vi "Tektronix TTR500 Series Calibration.vi"(11 "VISA resource name":refnum<visa-resource-name>="TCPIP0::localhost::5026::SOCKET") -> (0 "error out":errorcluster, 3 "Trace":T1(graph))   [LabVIEW 2012]
uses:
  <instrlib>/Tektronix TTR500 Series/Tektronix TTR500 Series.lvlib
panel:
  in  "Measurement Parameters (S21)":u16(ring)=1 items=["S11", "S21", "S31", "S41", "S12", "S22", "S32", "S42", "S13", "S23", "S33", "S43", "S14", "S24", "S34", "S44", "A", "B", "C", "D", "R1", "R2", "R3", "R4", "AUX1", "AUX2", "TR", "T", "R"]
  in  "IF Bandwidth (10k [Hz])":dbl=10000.0 format="%#p"
  in  "Number of Measurement Points (201)":i32=201
  in  "Power Level (0)":dbl format="%#.3f"
  in  "Stop Frequency (4G [Hz])":dbl=4000000000.0 format="%#p"
  in  "Start Frequency (1G [Hz])":dbl=1000000000.0 format="%#p"
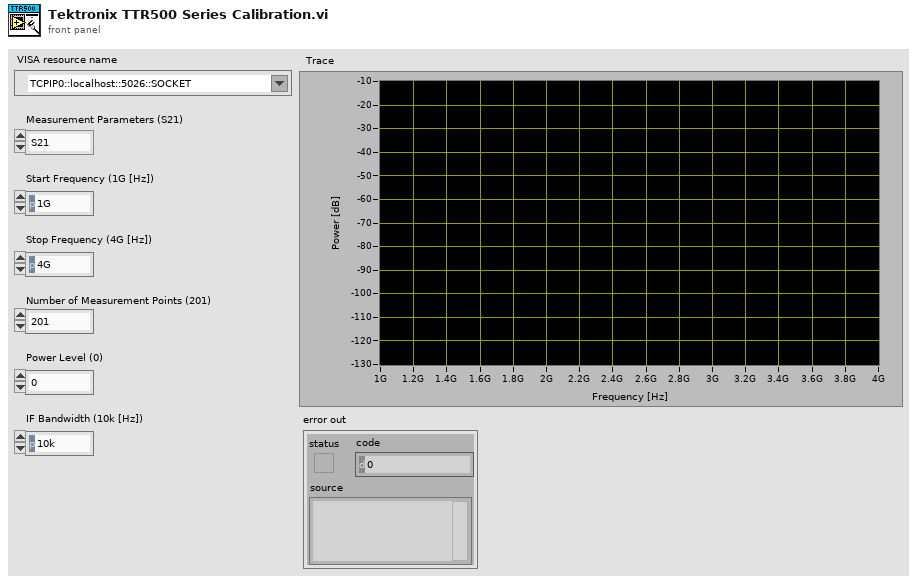
[diagram p1: front panel]
types:
  T1 = cluster{"Stimulus Data":dbl[], "Primary / Real":dbl[]}
  T2 = cluster{"Standard":u16, "Port 1 - response":i32, "Port 2 - stimulus":i32}[]
  T3 = enum16{"Open", "Short", "Load", "Through", "Isolation", "Gain Phase Open", "Gain Phase Short", "Gain Phase Load", "Gain Phase Through", "Gain Phase Isolation"}
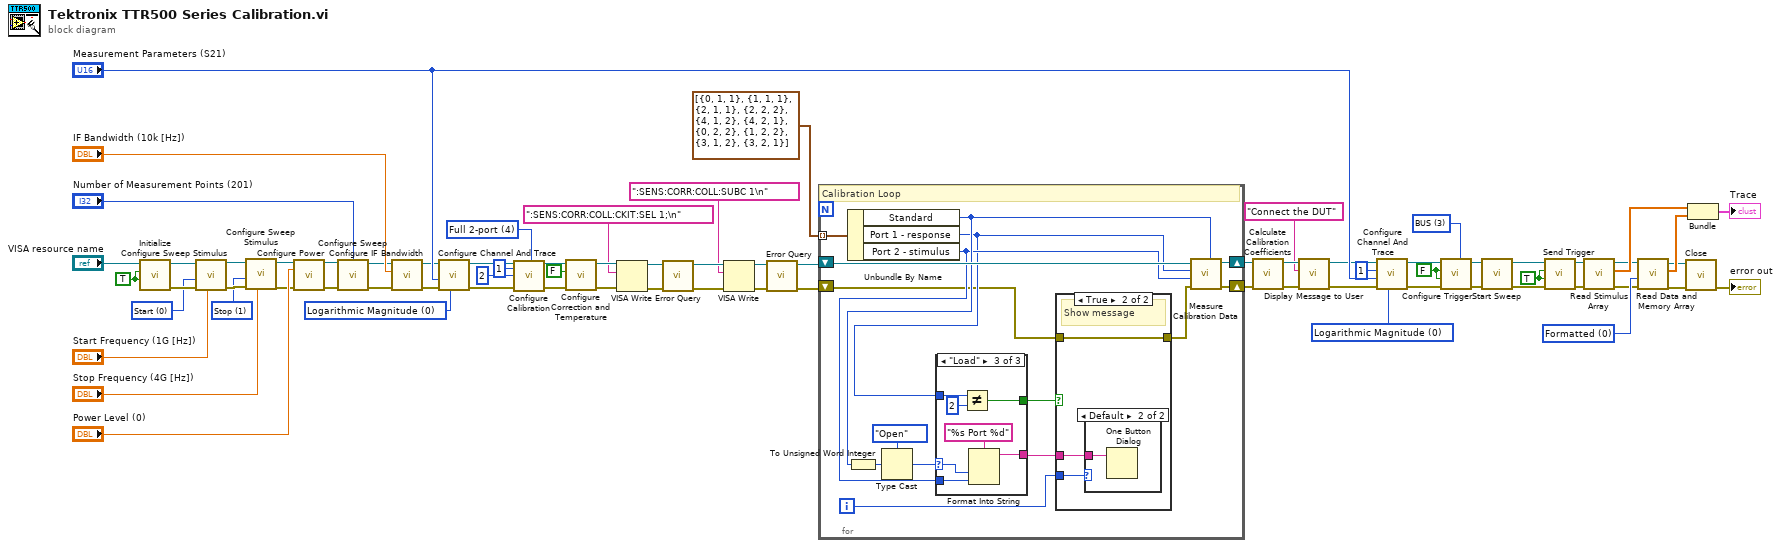
[diagram p0: block diagram]
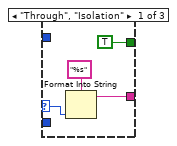
[diagram p2: hidden frame]
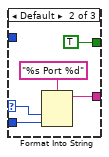
[diagram p3: hidden frame]
diagram:
  w34 = u16 4 items=["Open", "Short", "Through", "1-port", "Full 2-port", "Full 3-port", "Full 4-port", "Enhanced Response", "Gain Phase Open", "Gain Phase Short", "Gain Phase Through", "Gain Phase 1 port "] ("Calibration Type (6: Full 4-port)")
  w35 = u16 0 items=["Logarithmic Magnitude", "Phase", "Group Delay", "Smith Chart  Linear (Lin/Phase)", "Smith Chart  Logarithmic (Log/Phase)", "Smith Chart  Complex (Real/Imag)", "Smith Chart  Impedance (R+jX)", "Smith Chart  Admittance (G+jB)", "Polar Format (Linear)", "Polar Format (Logarithmic)", "Polar Format (Re/Im)", "Linear Magnitude", "SWR", "Real", "Imaginary", "Epanded Phase", "Positive Phase"] ("Data Format (0: Logarithmic Magnitude)")
  w44 = u16 1 items=["Start", "Stop", "Center", "Span"] ("Stimulus (0: Start)")
  w47 = u16 0 items=["Start", "Stop", "Center", "Span"] ("Stimulus (0: Start)")
  w57 = u16 0 items=["Formatted", "Corrected"] ("Correction (0: Data)")
  w49 = TRUE ("Wait for OPC (F: Do not Wait)")
  w58 = FALSE ("Continuous Sweep (T: Enable)")
  w60 = u16 3 items=["Internal", "External", "Manual", "BUS"] ("Trigger Source (0: Internal)")
  w63 = u16 0 items=["Logarithmic Magnitude", "Phase", "Group Delay", "Smith Chart  Linear (Lin/Phase)", "Smith Chart  Logarithmic (Log/Phase)", "Smith Chart  Complex (Real/Imag)", "Smith Chart  Impedance (R+jX)", "Smith Chart  Admittance (G+jB)", "Polar Format (Linear)", "Polar Format (Logarithmic)", "Polar Format (Re/Im)", "Linear Magnitude", "SWR", "Real", "Imaginary", "Epanded Phase", "Positive Phase"] ("Data Format (0: Logarithmic Magnitude)")
  w11 = TRUE ("Reset? (T: Yes)")
  n1 = call <instrlib>:"Initialize.vi"("Reset? (T: Yes)"=w11, "ID Query? (T: Yes)"=w11, "VISA resource name"="VISA resource name") -> ("error out"=w71:errorcluster, "VISA resource name out"=w70:refnum<visa-resource-name>)  [unwired: 6 in, 1 out]
  n2 = call <instrlib>:"Configure Sweep Stimulus.vi"("Parameter (0.0)"="Start Frequency (1G [Hz])", "error in (no error)"=w71, "Stimulus (0: Start)"=w47, "VISA resource name"=w70) -> ("error out"=w46:errorcluster, "VISA resource name out"=w45:refnum<visa-resource-name>)  [unwired: 6 in]
  n3 = call <instrlib>:"Configure Sweep Stimulus.vi"("Parameter (0.0)"="Stop Frequency (4G [Hz])", "error in (no error)"=w46, "Stimulus (0: Start)"=w44, "VISA resource name"=w45) -> ("error out"=w42:errorcluster, "VISA resource name out"=w43:refnum<visa-resource-name>)  [unwired: 6 in]
  n4 = call <instrlib>:"Configure Power.vi"("VISA resource name"=w43, "Power Level (0.0)"="Power Level (0)", "error in (no error)"=w42) -> ("VISA resource name out"=w41:refnum<visa-resource-name>, "error out"=w40:errorcluster)  [unwired: 11 in]
  n5 = call <instrlib>:"Configure Sweep.vi"("VISA resource name"=w41, "Number of Measurement Points (201)"="Number of Measurement Points (201)", "error in (no error)"=w40) -> ("VISA resource name out"=w39:refnum<visa-resource-name>, "error out"=w38:errorcluster)  [unwired: 11 in]
  n6 = call <instrlib>:"Configure IF Bandwidth.vi"("error in (no error)"=w38, "IF Bandwidth (100000.0)"="IF Bandwidth (10k [Hz])", "VISA resource name"=w39) -> ("error out"=w37:errorcluster, "VISA resource name out"=w36:refnum<visa-resource-name>)  [unwired: 7 in]
  n7 = call <instrlib>:"Configure Channel And Trace.vi"("Data Format (0: Logarithmic Magnitude)"=w35, "error in (no error)"=w37, "Measurement Parameters (0: S11)"="Measurement Parameters (S21)", "VISA resource name"=w36) -> ("error out"=w27:errorcluster, "VISA resource name out"=w28:refnum<visa-resource-name>)  [unwired: 6 in]
  n8 = call <instrlib>:"Configure Calibration.vi"("VISA resource name"=w28, "Port 1 (1)"=1, "Port 2 (1)"=2, "error in (no error)"=w27, "Calibration Type (4: Full 2-port)"=w34) -> ("VISA resource name out"=w30:refnum<visa-resource-name>, "error out"=w31:errorcluster)  [unwired: 13 in]
  n9 = call <instrlib>:"Configure Correction and Temperature.vi"("error in (no error)"=w31, "System Error Correction (T: Enable)"=FALSE, "VISA resource name"=w30) -> ("error out"=w25:errorcluster, "VISA resource name out"=w26:refnum<visa-resource-name>)  [unwired: 7 in]
  n10 = VISA Write(VISA resource name=w26, write buffer=":SENS:CORR:COLL:CKIT:SEL 1;\n" ("String ()"), error in (no error)=w25) -> (VISA resource name out=w19:refnum<visa-resource-name>, error out=w18:errorcluster)  [unwired: 1 out]
  n11 = call <instrlib>:"Error Query.vi"("error in (no error)"=w18, "VISA resource name"=w19) -> ("error out"=w15:errorcluster, "VISA resource name out"=w14:refnum<visa-resource-name>)  [unwired: 6 in, 2 out]
  n12 = VISA Write(VISA resource name=w14, write buffer=":SENS:CORR:COLL:SUBC 1\n" ("Command"), error in (no error)=w15) -> (VISA resource name out=w16:refnum<visa-resource-name>, error out=w17:errorcluster)  [unwired: 1 out]
  n13 = call <instrlib>:"Error Query.vi"("error in (no error)"=w17, "VISA resource name"=w16) -> ("error out"=w23:errorcluster, "VISA resource name out"=w24:refnum<visa-resource-name>)  [unwired: 6 in, 2 out]
  n14 = for {
    tunnel: T2 [{"Standard"=0, "Port 1 - response"=1, "Port 2 - stimulus"=1}, {"Standard"=1, "Port 1 - response"=1, "Port 2 - stimulus"=1}, {"Standard"=2, "Port 1 - response"=1, "Port 2 - stimulus"=1}, {"Standard"=2, "Port 1 - response"=2, "Port 2 - stimulus"=2}, {"Standard"=4, "Port 1 - response"=1, "Port 2 - stimulus"=2}, {"Standard"=4, "Port 1 - response"=2, "Port 2 - stimulus"=1}, {"Standard"=0, "Port 1 - response"=2, "Port 2 - stimulus"=2}, {"Standard"=1, "Port 1 - response"=2, "Port 2 - stimulus"=2}, {"Standard"=3, "Port 1 - response"=1, "Port 2 - stimulus"=2}, {"Standard"=3, "Port 1 - response"=2, "Port 2 - stimulus"=1}] -> [w86] mode=indexing
    shift-right: [w85] -> w21
    shift-left: w23 -> [w75]
    shift-right: [w73] -> w20
    shift-left: w24 -> [w87]
    i -> [w78]
    # "Calibration Loop"
    n15 = Unbundle By Name(w86) -> ("Standard"=w81:u16, "Port 1 - response"=w77:i32, "Port 2 - stimulus"=w80:i32)
    n16 = To Unsigned Word Integer(number=w81) -> (unsigned 16bit integer=w83:u16)
    n17 = Type Cast(type=T3."Open" ("Standard (0: Open)"), x=w83) -> (*(type *) &x=w79:T3)
    n18 = case shown="\"Load\"" w79 {
      selector: w79 -> [w90 w93 w100]
      tunnel: [w91 w95 w102] -> w84
      tunnel: w80 -> [_ w94 w101]
      tunnel: w77 -> [_ _ w99]
      tunnel: [TRUE TRUE w97] -> w76
      frame "Through", "Isolation" {
        n19 = Format Into String(format string="%s", w90) -> (resulting string=w91:string)  [unwired: 2 in, 1 out]
      }
      frame Default {
        n20 = Format Into String(format string="%s Port %d", w93, w94) -> (resulting string=w95:string)  [unwired: 2 in, 1 out]
      }
      frame "Load" {
        n21 = Not Equal?(x=w99, y=2) -> (x != y?=w97:bool)
        n22 = Format Into String(format string="%s Port %d", w100, w101) -> (resulting string=w102:string)  [unwired: 2 in, 1 out]
      }
    }
    n23 = case shown="True" w76 {
      tunnel: w84 -> [_ w107]
      tunnel: w78 -> [_ w106]
      tunnel: w75 -> [w104 w105]
      tunnel: [w104 w105] -> w74
      frame False {
      }
      frame True {
        # "Show message"
        n24 = case shown="Default" w106 {
          tunnel: w107 -> [_ w108]
          frame 5, 9 {
          }
          frame Default {
            n25 = One Button Dialog(message=w108) -> ()  [unwired: 1 in, 1 out]
          }
        }
      }
    }
    n26 = call <instrlib>:"Measure Calibration Data.vi"("Standard (0: Open)"=w81, "error in (no error)"=w74, "Port 2 - stimulus (2)"=w80, "Port 1 - response (1)"=w77, "VISA resource name"=w87) -> ("error out"=w85:errorcluster, "VISA resource name out"=w73:refnum<visa-resource-name>)  [unwired: 5 in]
  }
  n27 = call <instrlib>:"Calculate Calibration Coefficients.vi"("error in (no error)"=w21, "VISA resource name"=w20) -> ("error out"=w4:errorcluster, "VISA resource name out"=w2:refnum<visa-resource-name>)  [unwired: 8 in]
  n28 = call "Display Message to User"("error in (no error)"=w4, "Message"="Connect the DUT") -> ("error out"=w3:errorcluster)  [unwired: 8 in, 1 out]
  n29 = call <instrlib>:"Configure Channel And Trace.vi"("Data Format (0: Logarithmic Magnitude)"=w63, "error in (no error)"=w3, "Measurement Parameters (0: S11)"="Measurement Parameters (S21)", "Number of Traces (1)"=1, "VISA resource name"=w2) -> ("error out"=w62:errorcluster, "VISA resource name out"=w61:refnum<visa-resource-name>)  [unwired: 5 in]
  n30 = call <instrlib>:"Configure Trigger.vi"("Trigger Source (0: Internal)"=w60, "error in (no error)"=w62, "Point Trigger (F: Disable)"=w58, "Continuous Sweep (T: Enable)"=w58, "VISA resource name"=w61) -> ("error out"=w53:errorcluster, "VISA resource name out"=w51:refnum<visa-resource-name>)  [unwired: 5 in]
  n31 = call <instrlib>:"Start Sweep.vi"("error in (no error)"=w53, "VISA resource name"=w51) -> ("error out"=w52:errorcluster, "VISA resource name out"=w50:refnum<visa-resource-name>)  [unwired: 8 in]
  n32 = call <instrlib>:"Send Trigger.vi"("error in (no error)"=w52, "Wait for OPC (F: Do not Wait)"=w49, "Ignore Trigger Source (F: Do not Ignore)"=w49, "VISA resource name"=w50) -> ("error out"=w9:errorcluster, "VISA resource name out"=w10:refnum<visa-resource-name>)  [unwired: 6 in]
  n33 = call <instrlib>:"Read Stimulus Array.vi"("error in (no error)"=w9, "VISA resource name"=w10) -> ("error out"=w7:errorcluster, "Stimulus Data"=w56:dbl[], "VISA resource name out"=w8:refnum<visa-resource-name>)  [unwired: 7 in]
  n34 = call <instrlib>:"Read Data and Memory Array.vi"("error in (no error)"=w7, "Correction (0: Data)"=w57, "VISA resource name"=w8) -> ("error out"=w5:errorcluster, "Primary / Real"=w55:dbl[], "VISA resource name out"=w6:refnum<visa-resource-name>)  [unwired: 5 in, 1 out]
  n35 = call <instrlib>:"Close.vi"("error in (no error)"=w5, "VISA resource name"=w6) -> ("error out"=→"error out":errorcluster)  [unwired: 9 in]
  n36 = Bundle("Stimulus Data"=w56, "Primary / Real"=w55) -> (→"Trace":T1)  [unwired: 1 in]
